vi "总磷单步调试对话框.vi"() -> ()   [LabVIEW 2016, in "斯坦道总磷总氮.lvlib"]
panel:
  in  "单步调试":T8={"注射泵"=enum."注入", "阀口选择"=enum."V1", "灯"=enum."未选择", "ADC值"=enum."未选择", "数值"=4000, "项目输入"=0, "控温"={"氨氮控温"=FALSE, "消解"=FALSE, "恒温"=FALSE, "降温"=FALSE}, "外设选择"={"蠕动泵"=FALSE, "电磁阀1"=FALSE, "电磁阀2"=FALSE, "慢速"=FALSE}, "外设选择2"={"V9-1"=FALSE, "V9-2"=FALSE, "顺时针"=FALSE, "逆时针"=FALSE}} {"项目输入" items=["总磷"=1, "总氮"=2, "氨氮"=3, "磷酸盐"=4, "硝氮"=5, "亚硝氮"=6, "硅酸盐"=7, "硫化物"=8, "CODcr"=22, "氟化物"=50]}
  in  "停止":bool
  out "注射器温度":sgl
  out "消解温度":sgl
  out "ADC":sgl
  out "F3":sgl format="%#.6f"
  out "F2":sgl format="%#.6f"
  out "F1":sgl format="%#.6f"
  out "F0":sgl format="%#.6f"
  in  "退出":bool
  in  "启动":bool
  # "单步调试界面"
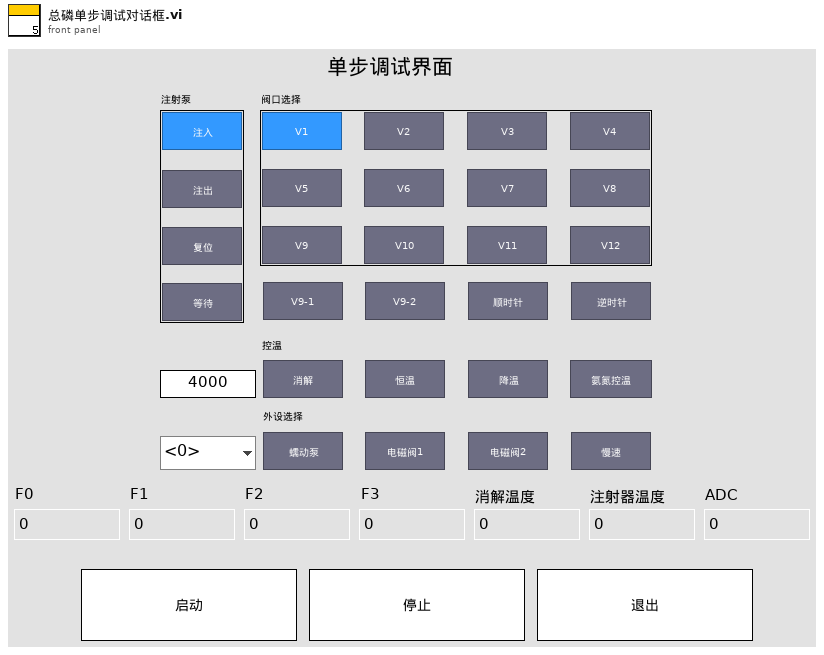
[diagram p1: front panel]
types:
  T1 = typedef "SingleStepTestV3.lvlib/SingleStepTestV3.lvclass/注射泵操作.ctl" = enum32{"复位", "注入", "注出", "等待"}
  T2 = typedef "SingleStepTestV3.lvlib/SingleStepTestV3.lvclass/阀口操作.ctl" = enum32{"未选择", "V1", "V2", "V3", "V4", "V5", "V6", "V7", "V8", "V9", "V10", "V11", "V12"}
  T3 = typedef "SingleStepTestV3.lvlib/SingleStepTestV3.lvclass/灯选择.ctl" = enum32{"未选择", "365", "520", "660", "氙灯/紫灯"}
  T4 = typedef "SingleStepTestV3.lvlib/SingleStepTestV3.lvclass/ADC选择.ctl" = enum32{"未选择", "ADC365", "ADC520", "ADC660", "光谱仪"}
  T5 = typedef "SingleStepTestV3.lvlib/SingleStepTestV3.lvclass/控温操作.ctl" = cluster{"氨氮控温":bool, "消解":bool, "恒温":bool, "降温":bool}
  T6 = typedef "SingleStepTestV3.lvlib/SingleStepTestV3.lvclass/外设选择.ctl" = cluster{"蠕动泵":bool, "电磁阀1":bool, "电磁阀2":bool, "慢速":bool}
  T7 = typedef "SingleStepTestV3.lvlib/SingleStepTestV3.lvclass/外设选择2.ctl" = cluster{"V9-1":bool, "V9-2":bool, "顺时针":bool, "逆时针":bool}
  T8 = cluster{"注射泵":T1, "阀口选择":T2, "灯":T3, "ADC值":T4, "数值":i16, "项目输入":u16, "控温":T5, "外设选择":T6, "外设选择2":T7}
  T9 = typedef "SingleStepTestV3.lvlib/SingleStepTestV3.lvclass/仪器版本.ctl" = enum16{"A版", "B版", "A1版"}
  T10 = typedef "操作日志字段定义.ctl" = cluster{"时间":timestamp, "参数":string, "日志信息":string, "流程参数":string}
  T11 = cluster{"系统时间":timestamp, "工作状态":u16, "测量模式":enum16{"待机", "连续模式", "周期模式", "定点模式", "受控模式", "手动模式"}, "告警代码":u16, "故障代码":u16, "日志代码":u16, "软件版本":u16, "F0":sgl, "F1":sgl, "F2":sgl, "F3":sgl, "T":sgl, "H":sgl, "id":u16, "flowid":u16, "量程":u16, "总磷控温温度1":sgl, "营养盐控温温度2":sgl, "ADC":sgl}
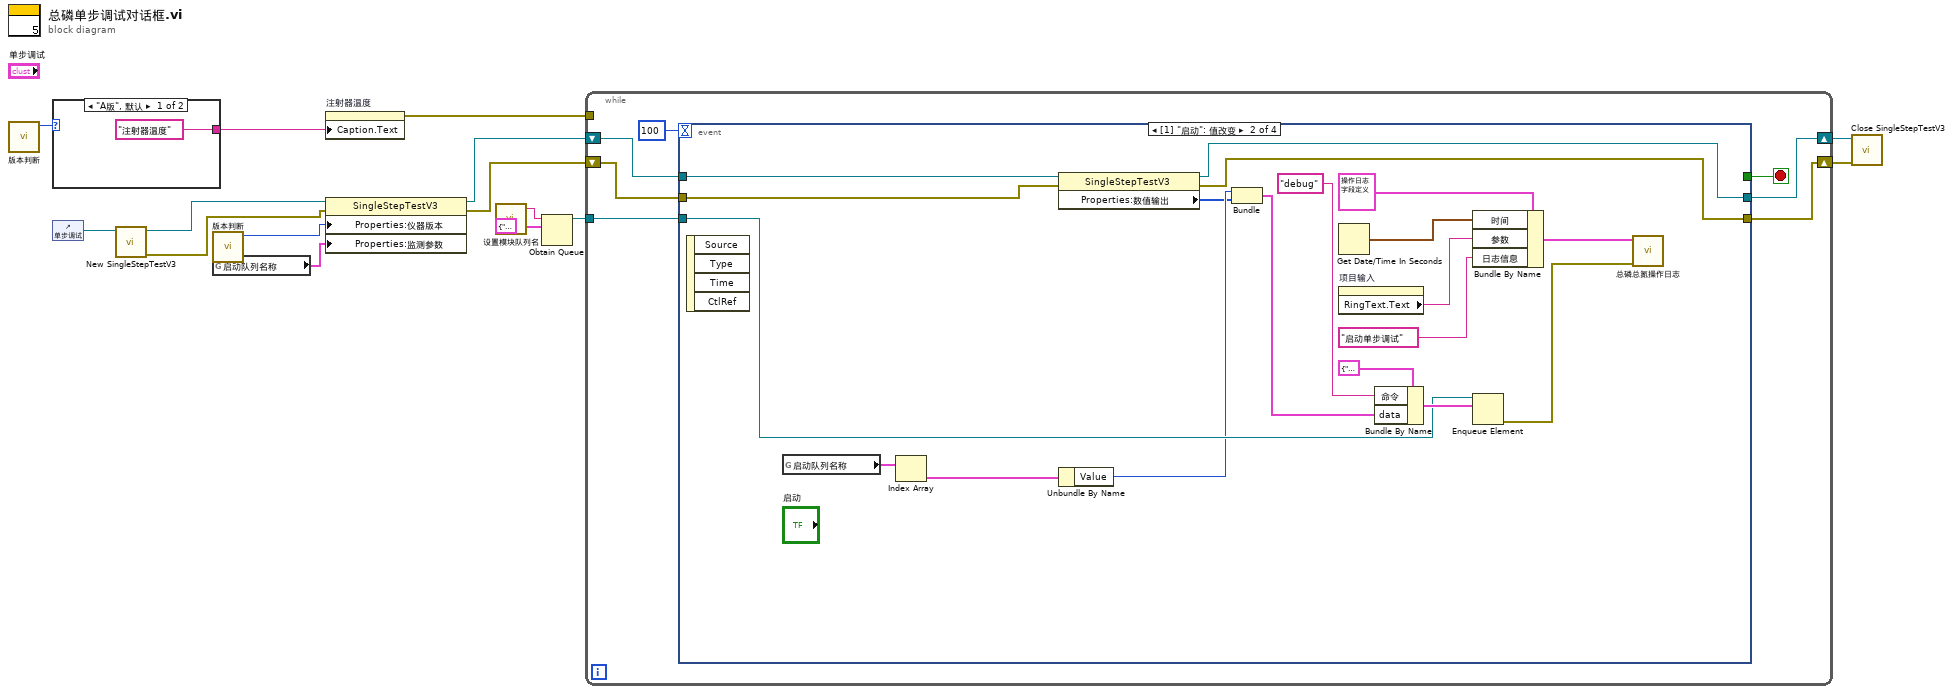
[diagram p0: block diagram]
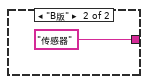
[diagram p2: hidden frame]
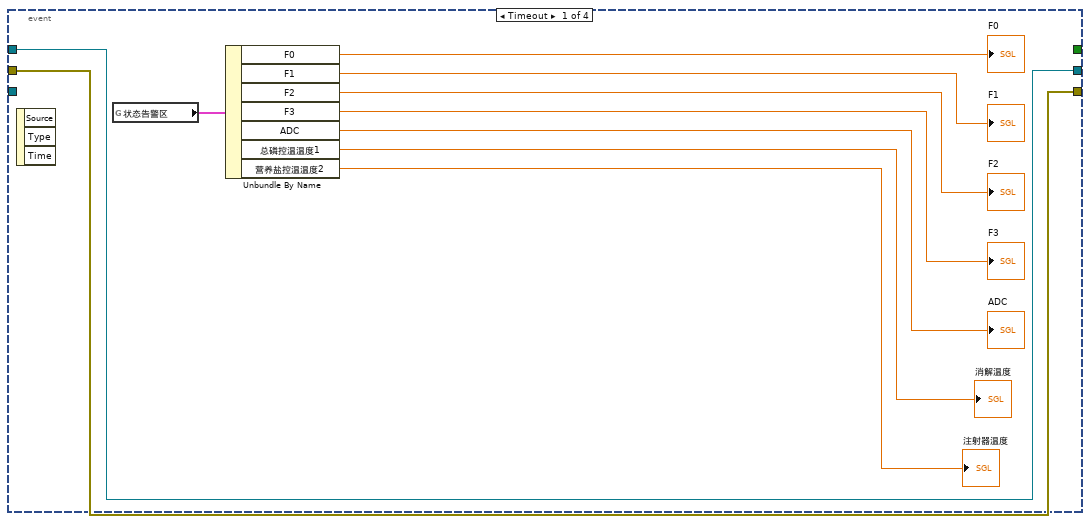
[diagram p3: hidden frame]
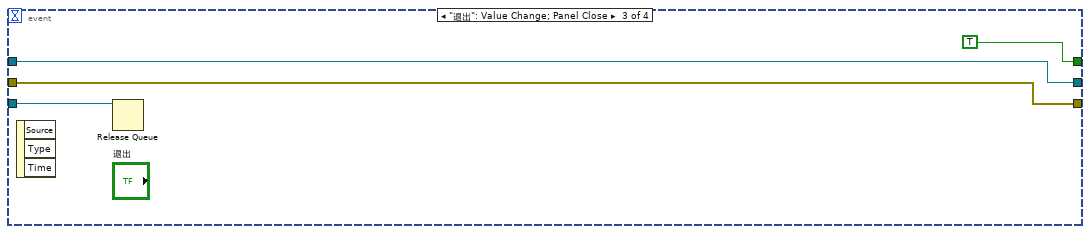
[diagram p4: hidden frame]
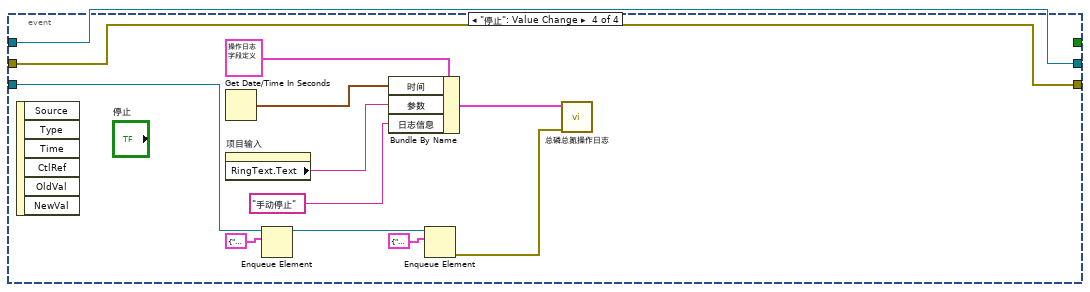
[diagram p5: hidden frame]
diagram:
  n1 = call "版本判断.vi"() -> ("仪器版本"=w12:T9)  [unwired: 11 in]
  n2 = case shown="\"A版\", 默认" w12 {
    tunnel: ["注射器温度" ("标题.文本") "传感器" ("标题.文本")] -> w11
    frame "A版", Default {
    }
    frame "B版" {
    }
  }
  n3 = control-ref of="单步调试"() -> (w7:refnum<vi>)
  n4 = call "New SingleStepTestV3.vi"("Reference"=w7) -> ("error out"=w4:errorcluster, "SingleStepTestV3 out"=w3:refnum<class "SingleStepTestV3.lvclass">)  [unwired: 9 in]
  n5 = call "版本判断.vi"() -> ("仪器版本"=w2:T9)  [unwired: 11 in]
  n6 = global read "model config var.vi" "启动队列名称"() -> (w1:cluster{"String":string, "Value":u16}[])
  n7 = property on="注射器温度" class="DigNum (严格)"("Caption.Text"=w11) -> (error out=w10:errorcluster)  [unwired: 2 in, 1 out]
  n8 = property class="SingleStepTestV3"(reference=w3, error in=w4, "Properties:仪器版本"=w2, "Properties:监测参数"=w1) -> (reference out=w9:refnum<class "SingleStepTestV3.lvclass">, error out=w8:errorcluster)
  n9 = call "设置模块队列名.vi"() -> ("Msg"=w13:string)  [unwired: 5 in]
  n10 = Obtain Queue(name (unnamed)=w13, element data type=cluster{"命令":string, "data":variant} {"命令"="", "data"=variant}) -> (queue out=w14:refnum<queue>)  [unwired: 3 in, 2 out]
  n11 = while {
    tunnel: w14 -> [w24]
    tunnel: w10 -> [_]
    shift-right: [w18] -> w5
    shift-left: w8 -> [w20]
    shift-right: [w19] -> w6
    shift-left: w9 -> [w21]
    stop <- w23 stop-if-true
    n12 = event shown="[1] \"启动\": 值改变" {
      selector: _ -> [_ _ _ _]
      dyn-events: _ -> [_ _ _ _]
      timeout: 100 -> [_ _ _ _]
      tunnel: w24 -> [_ w49 w56 w66]
      tunnel: [_ _ TRUE _] -> w23
      tunnel: w21 -> [w26 w45 w55 w65]
      tunnel: w20 -> [w25 w44 w54 w64]
      tunnel: [w26 w41 w55 w65] -> w19
      tunnel: [w25 w43 w54 w64] -> w18
      event Timeout {
        n13 = event-data() -> ()  [unwired: 1 in, 3 out]
        n14 = global read "VAR总磷总氮全局变量.vi" "状态告警区"() -> (w27:T11)
        n15 = Unbundle By Name(w27) -> ("F0"=→"F0":sgl, "F1"=→"F1":sgl, "F2"=→"F2":sgl, "F3"=→"F3":sgl, "ADC"=→"ADC":sgl, "总磷控温温度1"=→"消解温度":sgl, "营养盐控温温度2"=→"注射器温度":sgl)
      }
      event "启动": Value Change {
        n16 = event-data() -> ()  [unwired: 1 in, 4 out]
        n17 = global read "model config var.vi" "启动队列名称"() -> (w46:cluster{"String":string, "Value":u16}[])
        n18 = Index Array(array=w46) -> (element=w48:cluster{"String":string, "Value":u16})  [unwired: 1 in]
        n19 = property class="SingleStepTestV3"(reference=w45, error in=w44) -> (reference out=w41:refnum<class "SingleStepTestV3.lvclass">, error out=w43:errorcluster, "Properties:数值输出"=w42:u16[])
        n20 = Unbundle By Name(w48) -> ("Value"=w47:u16)
        n21 = Bundle("Value"=w47, "Properties:数值输出"=w42) -> (w50:cluster{"Value":u16, "Properties:数值输出":u16[]})  [unwired: 1 in]
        n22 = Get Date/Time In Seconds() -> (seconds since 1Jan1904=w38:timestamp)
        n23 = property on="项目输入" class="Ring (严格)"() -> ("RingText.Text"=w35:string)  [unwired: 2 in, 2 out]
        n24 = Bundle By Name(cluster=cluster{"命令":string, "data":variant} {"命令"="", "data"=variant} ("元素"), "命令"="debug", "data"=w50) -> (w51:cluster{"命令":string, "data":variant})
        n25 = Bundle By Name(cluster=T10 {"时间"=timestamp(0 s since 1904-01-01), "参数"="", "日志信息"="", "流程参数"=""} ("data in"), "时间"=w38, "参数"=w35, "日志信息"="启动单步调试") -> (w39:T10)
        n26 = Enqueue Element(queue=w49, element=w51) -> (error out=w36:errorcluster)  [unwired: 2 in, 2 out]
        n27 = call "总磷总氮操作日志.vi"("错误输入（无错误）"=w36, "data in"=w39) -> ()  [unwired: 9 in, 1 out]
      }
      event "退出": Value Change; Panel Close {
        n28 = event-data() -> ()  [unwired: 1 in, 3 out]
        n29 = Release Queue(queue=w56) -> ()  [unwired: 2 in, 3 out]
      }
      event "停止": Value Change {
        n30 = event-data() -> ()  [unwired: 1 in, 6 out]
        n31 = Get Date/Time In Seconds() -> (seconds since 1Jan1904=w61:timestamp)
        n32 = property on="项目输入" class="Ring (严格)"() -> ("RingText.Text"=w58:string)  [unwired: 2 in, 2 out]
        n33 = Enqueue Element(queue=w66, element=cluster{"命令":string, "data":variant} {"命令"="启动", "data"=variant(cluster{"站号":u16, "控制命令输出":u16[]} {"站号"=1, "控制命令输出"=[2816]})} ("元素")) -> (queue out=w67:refnum<queue>)  [unwired: 2 in, 2 out]
        n34 = Bundle By Name(cluster=T10 {"时间"=timestamp(0 s since 1904-01-01), "参数"="", "日志信息"="", "流程参数"=""} ("data in"), "时间"=w61, "参数"=w58, "日志信息"="手动停止") -> (w62:T10)
        n35 = Enqueue Element(queue=w67, element=cluster{"命令":string, "data":variant} {"命令"="启动", "data"=variant(cluster{"站号":u16, "控制命令输出":u16[]} {"站号"=2, "控制命令输出"=[2816]})} ("元素")) -> (error out=w59:errorcluster)  [unwired: 2 in, 2 out]
        n36 = call "总磷总氮操作日志.vi"("错误输入（无错误）"=w59, "data in"=w62) -> ()  [unwired: 9 in, 1 out]
      }
    }
  }
  n37 = call "Close SingleStepTestV3.vi"("error in (no error)"=w5, "SingleStepTestV3 in"=w6) -> ()  [unwired: 9 in, 1 out]
